vi "Insert Into Array (Multi Numeric).vi"(9 "index":i32, 10 "Array":dbl[](array[numeric]), 11 "JSON Value in":refnum<class "JSON Value.lvclass">) -> (3 "JSON Value out":refnum<class "JSON Value.lvclass">)   [LabVIEW 2016, in "JSON Value.lvclass"]
doc: "Inserts an element or subarray into a JSON array at the point you specify in index."
uses:
  JSON Value.lvclass
  Insert Into Array (Multi).vi
  New JSON Value/New JSON Numeric.vi
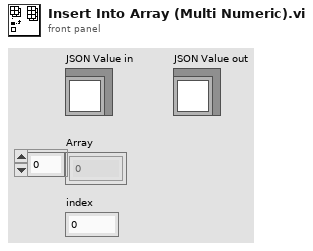
[diagram p1: front panel]
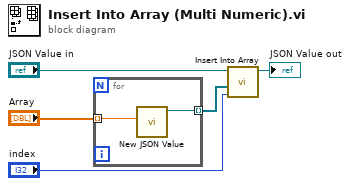
[diagram p0: block diagram]
diagram:
  n1 = for {
    tunnel: "Array" -> [w7] mode=indexing
    tunnel: [w6] -> w1 mode=indexing
    n2 = call-poly "New JSON Value.vi"("value"=w7) -> ("JSON Value out"=w6:refnum<class "JSON Value.lvclass">)  [unwired: 9 in, 1 out]
  }
  n3 = call-poly "Insert Into Array.vi"("index"="index", "Array"=w1, "JSON Array in"="JSON Value in") -> ("JSON Array out"=→"JSON Value out":refnum<class "JSON Value.lvclass">)  [unwired: 8 in]
